vi "WheelFeetToRotations.vi"(4 "feet":dbl) -> (1 "rotations":dbl)   [LabVIEW 2019]
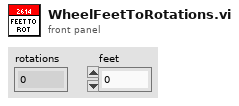
[diagram p1: front panel]
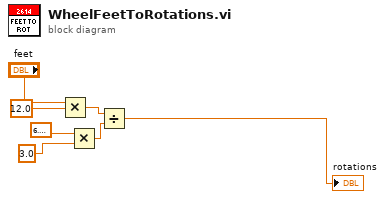
[diagram p0: block diagram]
diagram:
  n1 = Multiply(x="feet", y=12.0) -> (x*y=w5:dbl)
  n2 = Multiply(x=6.283185307179586, y=3.0) -> (x*y=w4:dbl)
  n3 = Divide(x=w5, y=w4) -> (x/y=→"rotations":dbl)
